vi "ReadWrite Channels.vi"(4 "ScheduledSDI":bool, 6 "Iteration":i32, 7 "Mode":T11, 8 "error in (no error)":errorcluster, 9 "hardware  in":T1, 10 "FIFOs In":T12, 11 "Channels In":T2[](array[typedef]) {"Labels Settings"."Driver Data"."Num Bits" min=1 max=32; "Labels Settings"."Driver Data"."Start Bit" min=8 max=31; "Labels Settings"."Block Data Refs"."Data Reference" format="%.0x"; "Labels Settings"."Label" format="%.0o"}) -> (0 "error out":errorcluster, 1 "hardware  out":T1, 2 "FIFOs Out":T12, 3 "Channels Out":T2[](array[typedef]) {"Labels Settings"."Driver Data"."Num Bits" min=1 max=32; "Labels Settings"."Driver Data"."Start Bit" min=8 max=31; "Labels Settings"."Block Data Refs"."Data Reference" format="%.0x"; "Labels Settings"."Label" format="%.0o"})   [LabVIEW 2011, in "AIT 1553 Custom Device.lvlib"]
uses:
  AIT 1553 Custom Device.lvlib
  RT Controls/FIFO.ctl
  RT Controls/ReadWrite Selector.ctl
  RT Controls/RT HW Channel.ctl
  RT Controls/RT Label Settings.ctl
  Controls and Global/Label.ctl
  Controls and Global/transferPeriod.ctl
  <vilib>/NI Veristand/Custom Device API/Block Data Reference.ctl
  <vilib>/NI Veristand/Custom Device API/Data Reference.ctl
  RT Controls/Driver Data.ctl
  Controls and Global/Start Bit.ctl
  Controls and Global/Number of Bits.ctl
  <userlib>/ARINC-429/vi/enum/Owl429HardwareSource.ctl
  <vilib>/NI Veristand/Custom Device API/NI VeriStand - Set Channel Values by Block Data Reference.vi
  Write outgoing label data.vi
  <vilib>/NI Veristand/Custom Device API/NI VeriStand - Get Channel Values by Block Data Reference.vi
  Read incoming label data.vi
  Double to selected bits.vi
  SubVIs/Word to double.vi
  <vilib>/NI Veristand/Custom Device API/Global Data Refs.vi
  <instrlib>/AIT 429/Public/Tx/Data/AIT 429 Set Scheduled Label Datum.vi
  <instrlib>/AIT 429/Public/Tx/Data/AIT 429 Get Scheduled Label Datum.vi
  <instrlib>/AIT 429/AIT 429.lvlib
  <userlib>/ARINC-429/Owl429.lvlib
  <vilib>/NI Veristand/Custom Device API/Custom Device API.lvlib
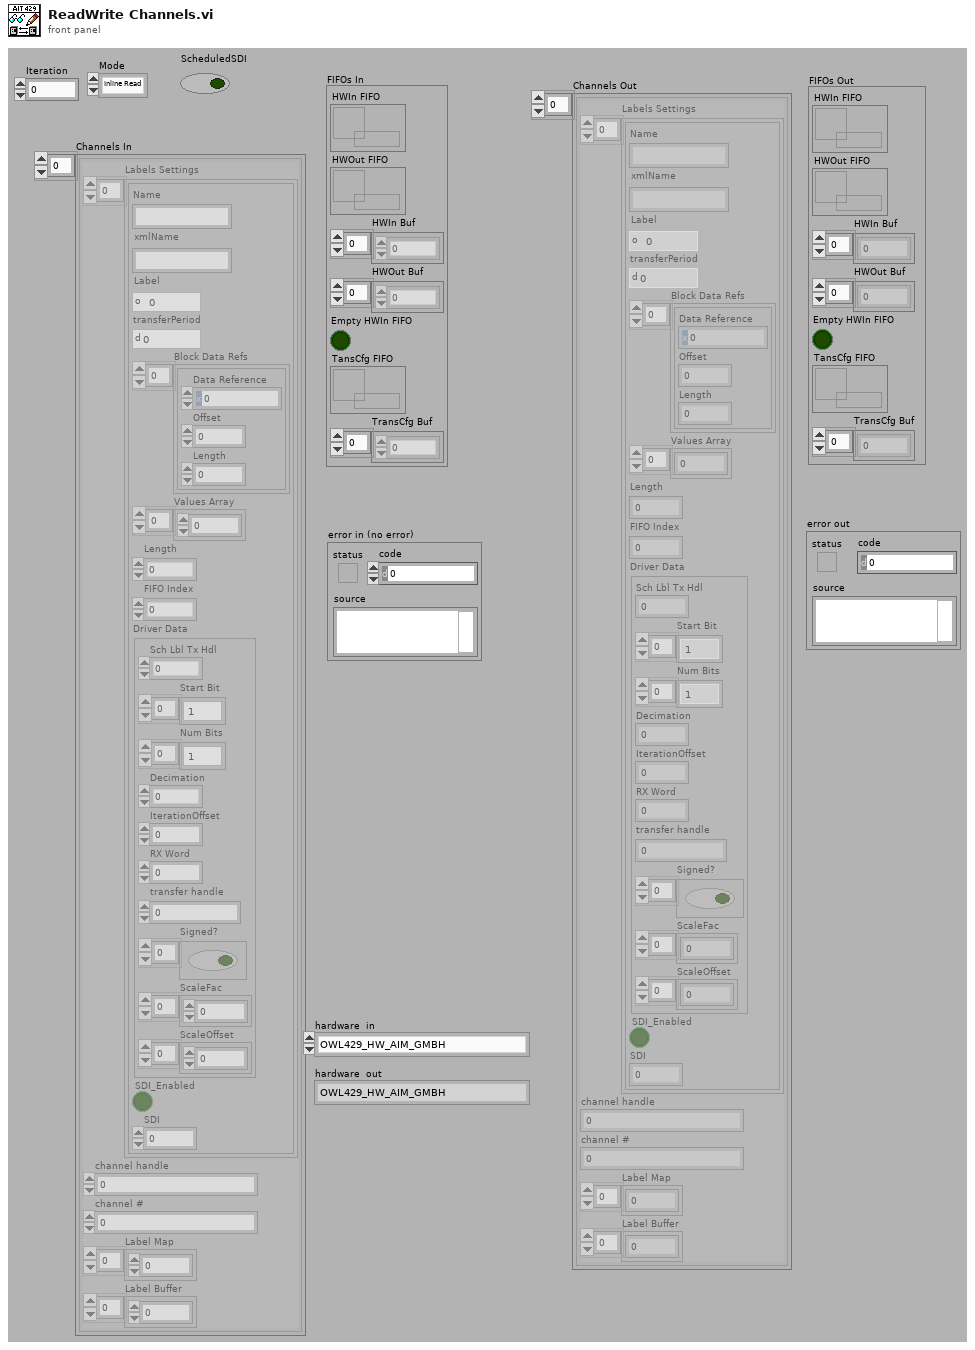
[diagram p1: front panel]
types:
  T1 = typedef "Owl429.lvlib/Owl429HardwareSource.ctl" = enum16{"OWL429_HW_AIM_GMBH", "OWL429_HW_AIT"}
  T2 = typedef "AIT 1553 Custom Device.lvlib/RT HW Channel.ctl" = cluster{"Labels Settings":T3[], "channel handle":u32, "channel #":u16, "Label Map":i32[], "Label Buffer":u32[]}
  T3 = typedef "AIT 1553 Custom Device.lvlib/RT Label Settings.ctl" = cluster{"Name":string, "xmlName":string, "Label":T4, "transferPeriod":T5, "Block Data Refs":T6[], "Values Array":dbl[], "Length":i32, "FIFO Index":i32, "Driver Data":T8, "SDI_Enabled":bool, "SDI":u8}
  T4 = typedef "AIT 1553 Custom Device.lvlib/Label.ctl" = u8
  T5 = typedef "AIT 1553 Custom Device.lvlib/transferPeriod.ctl" = u32
  T6 = typedef "Custom Device API.lvlib/Block Data Reference.ctl" = cluster{"Data Reference":T7, "Offset":i32, "Length":i32}
  T7 = typedef "Custom Device API.lvlib/Data Reference.ctl" = i32
  T8 = typedef "AIT 1553 Custom Device.lvlib/Driver Data.ctl" = cluster{"Sch Lbl Tx Hdl":u32, "Start Bit":T9[], "Num Bits":T10[], "Decimation":i32, "IterationOffset":i32, "RX Word":u32, "transfer handle":u32, "Signed?":bool[], "ScaleFac":dbl[], "ScaleOffset":dbl[]}
  T9 = typedef "AIT 1553 Custom Device.lvlib/Start Bit.ctl" = i32
  T10 = typedef "AIT 1553 Custom Device.lvlib/Number of Bits.ctl" = i32
  T11 = typedef "AIT 1553 Custom Device.lvlib/ReadWrite Selector.ctl" = enum16{"Inline Read", "Inline Write", "Async HWIn", "Async HWOut"}
  T12 = typedef "AIT 1553 Custom Device.lvlib/FIFO.ctl" = cluster{"HWIn FIFO":refnum<k33>, "HWOut FIFO":refnum<k33>, "HWIn Buf":dbl[], "HWOut Buf":dbl[], "Empty HWIn FIFO":bool, "TansCfg FIFO":refnum<k33>, "TransCfg Buf":dbl[]}
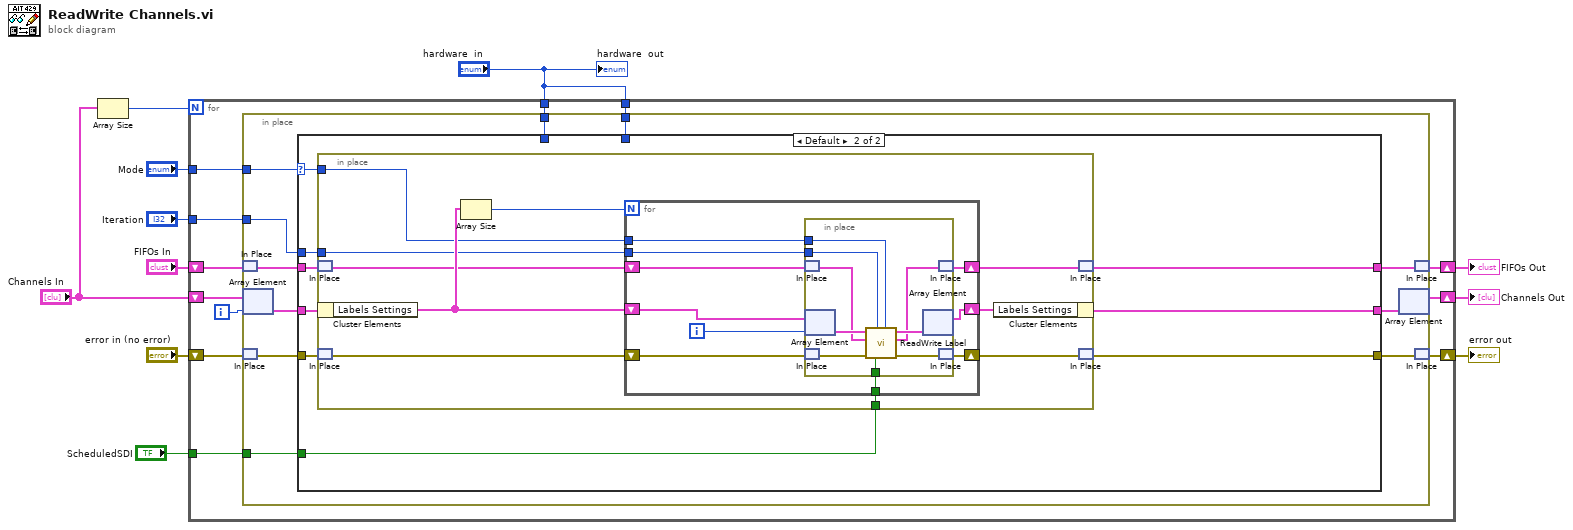
[diagram p0: block diagram]
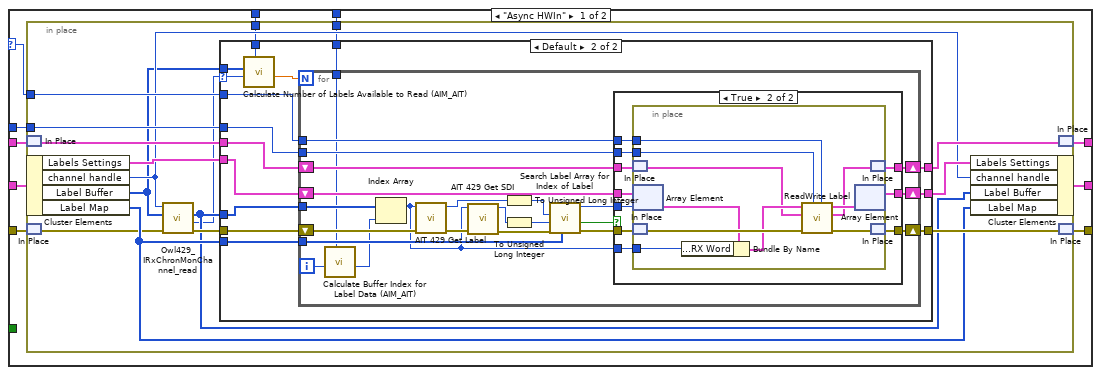
[diagram p2: hidden frame]
diagram:
  n1 = Array Size(array="Channels In") -> (size(s)=w4:i32)
  n2 = for {
    N: w4 -> [_]
    shift-right: [w19] -> w8
    shift-left: "error in (no error)" -> [w20]
    tunnel: "Mode" -> [w18]
    tunnel: "Iteration" -> [w15]
    shift-right: [w21] -> w6
    shift-left: "Channels In" -> [w23]
    shift-right: [w16] -> w11
    shift-left: "FIFOs In" -> [w17]
    tunnel: "hardware  in" -> [w14]
    tunnel: "hardware  in" -> [w13]
    tunnel: "ScheduledSDI" -> [w12]
    i -> [w22]
    n3 = in-place {
      in-place-border: w18 -> [w27]
      in-place-border: w15 -> [w28]
      in-place-border: w14 -> [w26]
      in-place-border: w13 -> [w25]
      in-place-border: w12 -> [w24]
      n4 = in-place-match #1(w17) -> (w30:T12)
      n5 = in-place-array #2(w23, w22) -> (w34:T2)
      n6 = in-place-match #3(w20) -> (w32:errorcluster)
      n7 = case shown="Default" w27 {
        selector: w27 -> [w37 w126]
        tunnel: w34 -> [w44 w133]
        tunnel: [w43 w132] -> w33
        tunnel: w32 -> [w42 w131]
        tunnel: [w41 w130] -> w31
        tunnel: w30 -> [w40 w129]
        tunnel: [w39 w128] -> w29
        tunnel: w28 -> [w38 w127]
        tunnel: w26 -> [w36 _]
        tunnel: w25 -> [w35 _]
        tunnel: w24 -> [_ w125]
        frame "Async HWIn" {
          n8 = in-place {
            in-place-border: w37 -> [w57]
            in-place-border: w38 -> [w55]
            in-place-border: w36 -> [w47]
            in-place-border: w35 -> [w46]
            n9 = in-place-match #4(w40) -> (w54:T12)
            n10 = in-place-cluster #5(w44) -> ("Labels Settings"=w60:T3[], "channel handle"=w50:u32, "Label Buffer"=w45:u32[], "Label Map"=w53:i32[])
            n11 = in-place-match #6(w42) -> (w51:errorcluster)
            n12 = call <userlib>:"Owl429_IRxChronMonChannel_read.vi"("error in (no error)"=w51, "data buffer"=w45, "channel handle"=w50) -> ("error out"=w52:errorcluster, "word count"=w48:u32, "data buffer"=w49:u32[])  [unwired: 5 in, 1 out]
            n13 = case shown="Default" w48 {
              selector: w48 -> [_ w67]
              tunnel: w60 -> [w62 w78]
              tunnel: [w62 w77] -> w59
              tunnel: [w63 w76] -> w58
              tunnel: w57 -> [_ w75]
              tunnel: [w61 w74] -> w56
              tunnel: w55 -> [_ w73]
              tunnel: w54 -> [w61 w72]
              tunnel: w53 -> [_ w71]
              tunnel: w52 -> [w63 w70]
              tunnel: w49 -> [_ w69]
              tunnel: w47 -> [_ w66]
              tunnel: w46 -> [_ w65]
              tunnel: w45 -> [_ w64]
              frame 0 {
              }
              frame Default {
                n14 = call "Calculate Number of Labels Available to Read (AIM_AIT).vi"("hardware  in"=w66, "entry count"=w67, "Label Buffer"=w64) -> ("# of labels available"=w68:dbl)  [unwired: 8 in]
                n15 = for {
                  N: w68 -> [_]
                  shift-right: [w100] -> w76
                  shift-left: w70 -> [w95]
                  tunnel: w75 -> [w99]
                  tunnel: w73 -> [w96]
                  tunnel: w69 -> [w91]
                  shift-right: [w97] -> w74
                  shift-left: w72 -> [w98]
                  shift-right: [w101] -> w77
                  shift-left: w78 -> [w94]
                  tunnel: w71 -> [w90]
                  tunnel: w65 -> [w86]
                  i -> [w88]
                  n16 = call "Calculate Buffer Index for Label Data (AIM_AIT).vi"("hardware  in"=w86, "Iteration"=w88) -> ("Buffer index"=w87:u32)  [unwired: 9 in]
                  n17 = Index Array(array=w91, index=w87) -> (element=w81:u32)
                  n18 = call <instrlib>:"AIT 429 Get Label.vi"("error in (no error)"=w95, "word"=w81) -> ("error out"=w85:errorcluster, "label"=w82:u8)  [unwired: 8 in]
                  n19 = call <instrlib>:"AIT 429 Get SDI.vi"("error in (no error)"=w85, "word"=w81) -> ("error out"=w83:errorcluster, "sdi"=w84:u8)  [unwired: 8 in]
                  n20 = To Unsigned Long Integer(number=w82) -> (unsigned 32bit integer=w80:u32)
                  n21 = To Unsigned Long Integer(number=w84) -> (unsigned 32bit integer=w79:u32)
                  n22 = call "Search Label Array for Index of Label.vi"("Label Map"=w90, "error in (no error)"=w83, "sdi"=w79, "label"=w80) -> ("error out"=w92:errorcluster, "Label Found?"=w89:bool, "Index"=w93:i32)  [unwired: 5 in]
                  n23 = case shown="True" w89 {
                    tunnel: [w103 w114] -> w101
                    tunnel: [w102 w113] -> w100
                    tunnel: w99 -> [_ w112]
                    tunnel: w98 -> [w104 w111]
                    tunnel: [w104 w110] -> w97
                    tunnel: w96 -> [_ w109]
                    tunnel: w94 -> [w103 w108]
                    tunnel: w93 -> [_ w107]
                    tunnel: w92 -> [w102 w106]
                    tunnel: w81 -> [_ w105]
                    frame False {
                    }
                    frame True {
                      n24 = in-place {
                        in-place-border: w112 -> [w118]
                        in-place-border: w109 -> [w117]
                        in-place-border: w105 -> [w119]
                        n25 = in-place-match #7(w111) -> (w116:T12)
                        n26 = in-place-array #8(w108, w107) -> (w122:T3)
                        n27 = in-place-match #9(w106) -> (w124:errorcluster)
                        n28 = Bundle By Name(cluster=w122, "Driver Data.RX Word"=w119) -> (w120:T3)
                        n29 = call "ReadWrite Label.vi"("Mode"=w118, "Iteration"=w117, "error in (no error)"=w124, "FIFOs In"=w116, "Label In"=w120) -> ("error out"=w123:errorcluster, "FIFOs Out"=w115:T12, "Label Out"=w121:T3)  [unwired: 4 in]
                        n30 = in-place-array #8(w121) -> (w114:T3[])  [unwired: 1 out]
                        n31 = in-place-match #7(w115) -> (w110:T12)
                        n32 = in-place-match #9(w123) -> (w113:errorcluster)
                      }
                    }
                  }
                }
              }
            }
            n33 = in-place-cluster #5("Labels Settings"=w59, "channel handle"=w50, "Label Buffer"=w49, "Label Map"=w53) -> (w43:T2)
            n34 = in-place-match #4(w56) -> (w39:T12)
            n35 = in-place-match #6(w58) -> (w41:errorcluster)
          }
        }
        frame Default {
          n36 = in-place {
            in-place-border: w126 -> [w139]
            in-place-border: w127 -> [w137]
            in-place-border: w125 -> [w134]
            n37 = in-place-match #10(w129) -> (w136:T12)
            n38 = in-place-cluster #11(w133) -> ("Labels Settings"=w142:T3[])
            n39 = in-place-match #12(w131) -> (w135:errorcluster)
            n40 = Array Size(array=w142) -> (size(s)=w143:i32)
            n41 = for {
              N: w143 -> [_]
              shift-right: [w149] -> w140
              shift-left: w135 -> [w150]
              tunnel: w139 -> [w148]
              tunnel: w137 -> [w145]
              shift-right: [w146] -> w138
              shift-left: w136 -> [w147]
              shift-right: [w151] -> w141
              shift-left: w142 -> [w153]
              tunnel: w134 -> [w144]
              i -> [w152]
              n42 = in-place {
                in-place-border: w148 -> [w159]
                in-place-border: w145 -> [w160]
                in-place-border: w144 -> [w154]
                n43 = in-place-match #13(w147) -> (w155:T12)
                n44 = in-place-array #14(w153, w152) -> (w156:T3)
                n45 = in-place-match #15(w150) -> (w157:errorcluster)
                n46 = call "ReadWrite Label.vi"("Mode"=w159, "ScheduledSDI"=w154, "Iteration"=w160, "error in (no error)"=w157, "FIFOs In"=w155, "Label In"=w156) -> ("error out"=w162:errorcluster, "FIFOs Out"=w158:T12, "Label Out"=w161:T3)  [unwired: 3 in]
                n47 = in-place-array #14(w161) -> (w151:T3[])  [unwired: 1 out]
                n48 = in-place-match #13(w158) -> (w146:T12)
                n49 = in-place-match #15(w162) -> (w149:errorcluster)
              }
            }
            n50 = in-place-cluster #11("Labels Settings"=w141) -> (w132:T2)
            n51 = in-place-match #10(w138) -> (w128:T12)
            n52 = in-place-match #12(w140) -> (w130:errorcluster)
          }
        }
      }
      n53 = in-place-array #2(w33) -> (w21:T2[])  [unwired: 1 out]
      n54 = in-place-match #1(w29) -> (w16:T12)
      n55 = in-place-match #3(w31) -> (w19:errorcluster)
    }
  }
  "FIFOs Out" <- w11
  "error out" <- w8
  "Channels Out" <- w6
  "hardware  out" <- "hardware  in"
